vi "FTW-KernelFilepath.vi"(8 "error in":errorcluster) -> (0 "error out":errorcluster, 1 "Library Version":string, 2 "Library Filepath":path)   [LabVIEW 2014]
uses:
  src/error/FTW-ERR-ThrowError.vi
  src/error/FTW-ERR-NoErrorConstant.vi
  src/error/FTW-ERR-CallChain.vi
  src/string/FTW-STR-ReplaceWhitespace.vi
  ftw32.dll
panel:
  # "Inputs"
  # "Outputs"
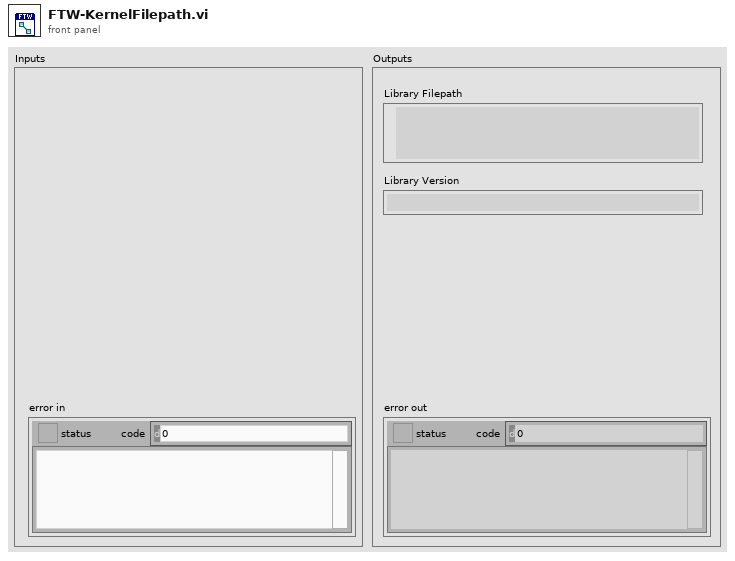
[diagram p1: front panel]
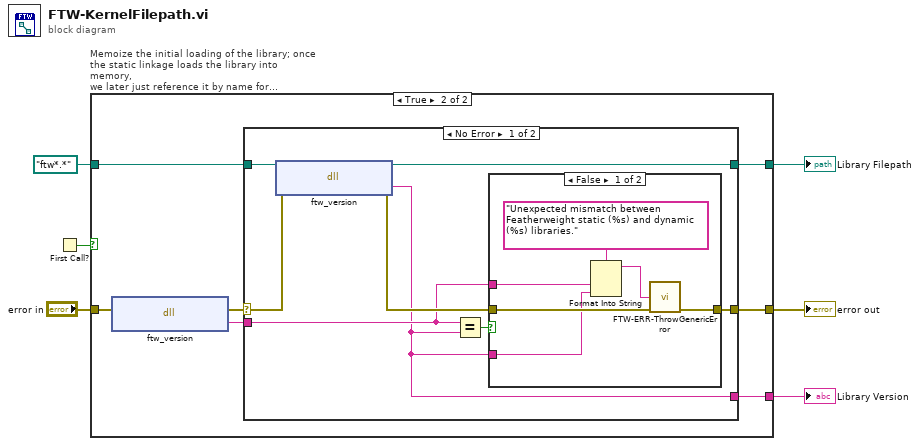
[diagram p0: block diagram]
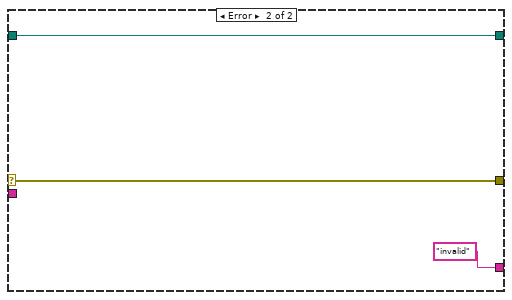
[diagram p4: hidden frame]
diagram:
  n1 = First Call?() -> (First Call?: T/F=w2:bool)
  n2 = case "Memoize the initial loading of the library; once the static linkage loads the library into memory,\nwe later just reference it by name for subsequent library method calls in this API" shown="True" w2 {
    tunnel: "error in" -> [w8 w13]
    tunnel: [_ w14] -> w4
    tunnel: [w8 w15] -> w5
    tunnel: path "ftw*.*" ("nanomsg Library Filepath") -> [w7 w10]
    tunnel: [w7 w9] -> w1
    frame False {
    }
    frame True {
      n3 = dll-call lib="C:/Users/Jack/repo/ftw-master/lib/ftw*.*" fn="ftw_version"(error in=w13) -> (error out=w11:errorcluster, "FTW Library Version"=w12:string)  [unwired: 2 in, 1 out]
      n4 = case shown="No Error" w11 {
        selector: w11 -> [w23 w32]
        tunnel: [w20 w32] -> w15
        tunnel: [w18 "invalid" ("Version (minus Build)")] -> w14
        tunnel: w10 -> [w17 w31]
        tunnel: w12 -> [w19 _]
        tunnel: [w16 w31] -> w9
        frame No Error {
          n5 = dll-call lib="?" fn="ftw_version"(path in=w17, error in=w23) -> (path out=w16:path, error out=w21:errorcluster, "FTW Library Version"=w18:string)  [unwired: 1 in]
          n6 = Equal?(x=w19, y=w18) -> (x = y?=w22:bool)
          n7 = case shown="False" w22 {
            tunnel: w21 -> [w29 w30]
            tunnel: [w28 w30] -> w20
            tunnel: w19 -> [w26 _]
            tunnel: w18 -> [w25 _]
            frame False {
              n8 = Format Into String(format string="Unexpected mismatch between Featherweight static (%s) and dynamic (%s) libraries.", w26, w25) -> (resulting string=w24:string)  [unwired: 2 in, 1 out]
              n9 = call "FTW-ERR-ThrowGenericError.vi"("Error Message"=w24, "error in"=w29) -> ("error out"=w28:errorcluster)  [unwired: 13 in]
            }
            frame True {
            }
          }
        }
        frame Error {
        }
      }
    }
  }
  "error out" <- w5
  "Library Filepath" <- w1
  "Library Version" <- w4
